vi "Reset.vi"(8 "error in (no error)":errorcluster, 10 "Reset":bool, 11 "ControlState in":T1 {"ChainMask" format="0x%02x"}) -> (0 "error out":errorcluster, 3 "ControlState out":T1 {"ChainMask" format="0x%02x"})   [LabVIEW 2023, in "ArduinoSerialBling.lvlib"]
uses:
  ArduinoSerialBling.lvlib
  ControlState.ctl
  ChainState.ctl
  TransmissionType.ctl
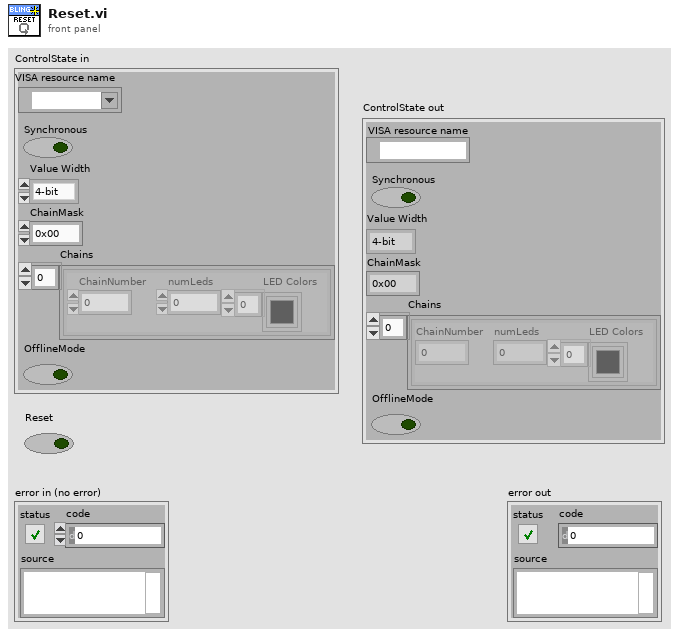
[diagram p1: front panel]
types:
  T1 = typedef "ArduinoSerialBling.lvlib/ControlState.ctl" = cluster{"VISA resource name":refnum<visa-resource-name>, "Synchronous":bool, "Value Width":enum16{"4-bit", "8-bit"}, "ChainMask":u8, "Chains":T2[], "OfflineMode":bool}
  T2 = typedef "ArduinoSerialBling.lvlib/ChainState.ctl" = cluster{"ChainNumber":u8, "numLeds":u8, "LED Colors":u32[]}
  T3 = typedef "ArduinoSerialBling.lvlib/TransmissionType.ctl" = enum16{"Follow Global", "Asynchronous", "Synchronous"}
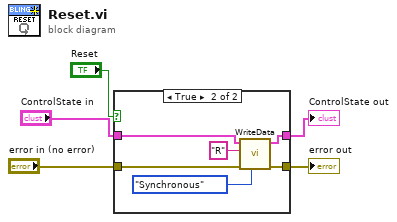
[diagram p0: block diagram]
diagram:
  n1 = case shown="True" "Reset" {
    tunnel: [w7 w9] -> w4
    tunnel: "error in (no error)" -> [w7 w10]
    tunnel: "ControlState in" -> [w6 w12]
    tunnel: [w6 w11] -> w1
    frame False {
    }
    frame True {
      n2 = call "WriteData.vi"("TransmissionType"=TransmissionType."Synchronous", "error in (no error)"=w10, "Command"="R" ("write buffer"), "ControlState in"=w12) -> ("error out"=w9:errorcluster, "ControlState out"=w11:T1)  [unwired: 4 in, 2 out]
    }
  }
  "error out" <- w4
  "ControlState out" <- w1
